vi "Local Test.vi"() -> ()   [LabVIEW 2021]
uses:
  Source/Omni-Bus/Omni_Bus.lvclass
  Source/Local Vars/Local Vars.lvclass
  Source/Omni-Bus/Support/Broad Types.ctl
  <vilib>/TSA/Abstract Data Classes/Constants/Support/U8/U8.vi
  <vilib>/TSA/Abstract Data Classes/Constants/Support/U8/Const_U8.lvclass
  <vilib>/TSA/Abstract Data Classes/Constants/Support/Str/Str.vi
  <vilib>/TSA/Abstract Data Classes/Constants/Support/Str/Const_Str.lvclass
  <vilib>/TSA/Abstract Data Classes/Constants/Support/DBL/DBL.vi
  <vilib>/TSA/Abstract Data Classes/Constants/Support/DBL/Const_DBL.lvclass
  <vilib>/TSA/Abstract Data Classes/Constants/Support/Bool/Bool.vi
  <vilib>/TSA/Abstract Data Classes/Constants/Support/Bool/Const_Bool.lvclass
  Source/Omni-Bus/Get/Static/Get Static Boolean.vi
  <vilib>/TSA/Abstract Data Classes/Abs_Types/Boolean/Static Read.vi
  <vilib>/TSA/Abstract Data Classes/Abs_Types/Boolean/Abs_Boolean.lvclass
  <vilib>/TSA/Abstract Data Classes/Abs_Types/Boolean/Static Write.vi
  C:/Program Files (x86)/National Instruments/LabVIEW 2021/vi.lib/TSA/Abstract Data Classes/Abs_Types/Value/Abs_Value.lvclass
  C:/Program Files (x86)/National Instruments/LabVIEW 2021/vi.lib/TSA/Abstract Data Classes/Abs_Types/Type/Abs_Type.lvclass
  C:/Program Files (x86)/National Instruments/LabVIEW 2021/vi.lib/TSA/Abstract Data Classes/Abs_Types/Boolean/Abs_Boolean.lvclass
  C:/Program Files (x86)/National Instruments/LabVIEW 2021/vi.lib/TSA/Abstract Data Classes/Abs_Types/Double Float/Abs_Double Float.lvclass
  C:/Program Files (x86)/National Instruments/LabVIEW 2021/vi.lib/TSA/Abstract Data Classes/Abs_Types/Floating Point/Abs_Floating Point.lvclass
  C:/Program Files (x86)/National Instruments/LabVIEW 2021/vi.lib/TSA/Abstract Data Classes/Abs_Types/Numeric/Abs_Numeric.lvclass
  C:/Program Files (x86)/National Instruments/LabVIEW 2021/vi.lib/TSA/Abstract Data Classes/Constants/Support/DBL/Const_DBL.lvclass
  C:/Program Files (x86)/National Instruments/LabVIEW 2021/vi.lib/TSA/Abstract Data Classes/Constants/Support/Interface/Const_Intf.lvclass
  <vilib>/TSA/Abstract Data Classes/Abs_Types/String/Abs_String.lvclass
  C:/Program Files (x86)/National Instruments/LabVIEW 2021/vi.lib/TSA/Abstract Data Classes/Abs_Types/String/Abs_String.lvclass
  C:/Program Files (x86)/National Instruments/LabVIEW 2021/vi.lib/TSA/Abstract Data Classes/Abs_Types/U8 Integer/Abs_U8 Integer.lvclass
  C:/Program Files (x86)/National Instruments/LabVIEW 2021/vi.lib/TSA/Abstract Data Classes/Abs_Types/Integer/Abs_Integer.lvclass
  C:/Program Files (x86)/National Instruments/LabVIEW 2021/vi.lib/TSA/Abstract Data Classes/Constants/Support/U8/Const_U8.lvclass
  <vilib>/TSA/Abstract Data Classes/Abs_Types/Value/Abs_Value.lvclass
  C:/Users/Tim/Documents/GitHub/VarBus/Source/Bus_Access/Bus_Access.lvclass
  C:/Users/Tim/Documents/GitHub/VarBus/Source/Local Vars/Local Vars.lvclass
  <vilib>/TSA/Abstract Data Classes/Abs_Types/Double Float/Support/Type.ctl
  <vilib>/TSA/Abstract Data Classes/Abs_Types/Double Float/Abs_Double Float.lvclass
panel:
  in  "Value 2":T1
  in  "stop 2":bool
  in  "stop":bool
  out "Value":T1
  out "Tags":string[](array[string])
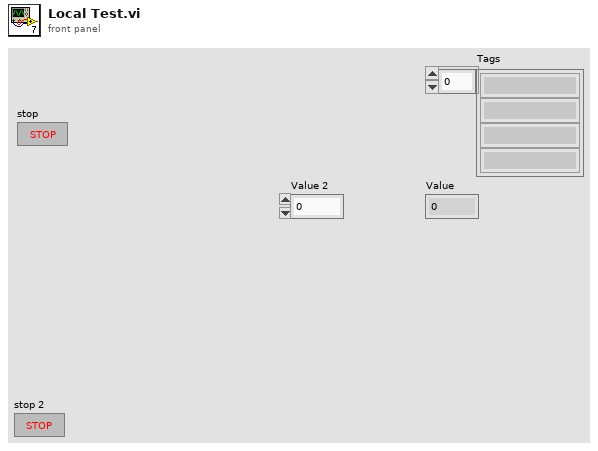
[diagram p1: front panel]
types:
  T1 = typedef "Abs_Double Float.lvclass/Type.ctl" = dbl
  T2 = typedef "Omni_Bus.lvclass/Broad Types.ctl" = enum16{"All Tags", "NI Specific Type", "Boolean", "String", "Numeric", "Float", "Integer", "Collection", "All Value Types", "Non Value Types"}
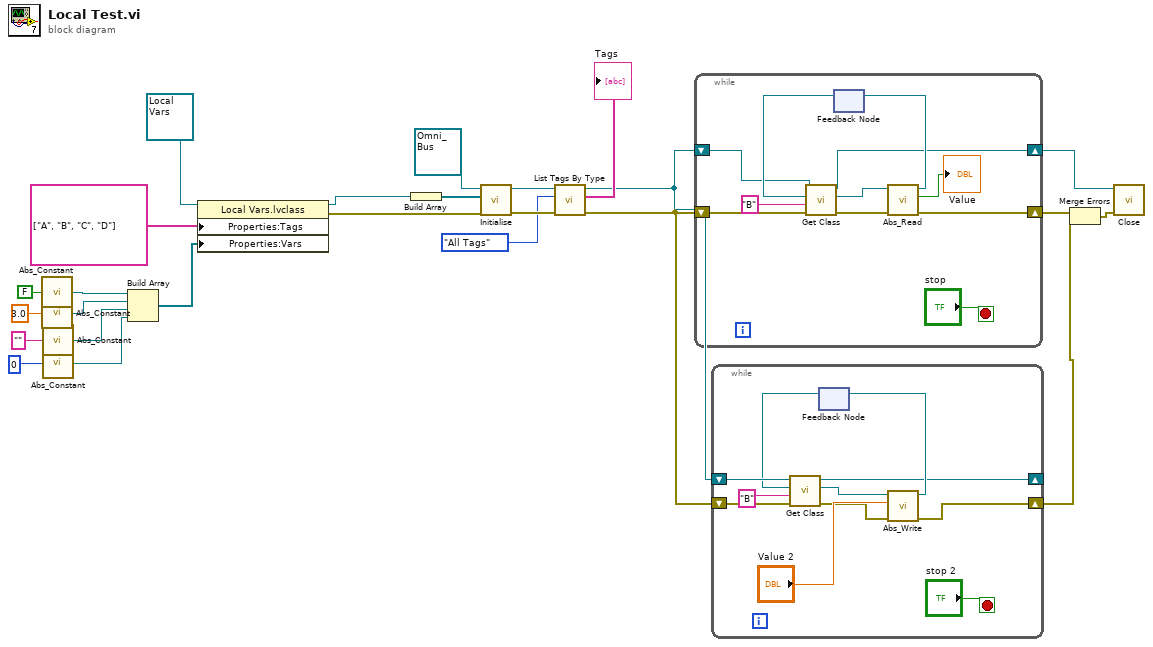
[diagram p0: block diagram]
diagram:
  n1 = call-poly <vilib>:"Abs_Constant.vi"("Boolean"=FALSE) -> ("Abs_Boolean.lvclass"=w19:refnum<class "Abs_Boolean.lvclass">)  [unwired: 4 in]
  n2 = call-poly <vilib>:"Abs_Constant.vi"("Value"=3.0) -> ("Constant"=w18:refnum<class "Const_DBL.lvclass">)  [unwired: 4 in]
  n3 = call-poly <vilib>:"Abs_Constant.vi"("String"="") -> ("Abs_String.lvclass"=w17:refnum<class "Abs_String.lvclass">)  [unwired: 4 in]
  n4 = call-poly <vilib>:"Abs_Constant.vi"("Value"=u8 0) -> ("Constant"=w9:refnum<class "Const_U8.lvclass">)  [unwired: 4 in]
  n5 = Build Array(w19, w18, w17, w9) -> (w14:refnum<class "Abs_Value.lvclass">[])
  n6 = property class="Local Vars.lvclass"(reference=refnum<class "Local Vars.lvclass"> refnum ("Data in"), "Properties:Tags"=string[] ["A", "B", "C", "D"] ("Tags"), "Properties:Vars"=w14) -> (reference out=w22:refnum<class "Local Vars.lvclass">, error out=w23:errorcluster)  [unwired: 1 in]
  n7 = Build Array(w22) -> (w24:refnum<class "Local Vars.lvclass">[])
  n8 = call-dynamic "Initialise.vi"("error in (no error)"=w23, "Var Access"=w24, "Var Bus in"=refnum<class "Omni_Bus.lvclass"> refnum) -> ("error out"=w12:errorcluster, "Var Bus out"=w13:refnum<class "Omni_Bus.lvclass">)  [unwired: 7 in]
  n9 = call-dynamic "List Tags By Type.vi"("error in (no error)"=w12, "Broad Types"=Broad_Types."All Tags", "Var Bus in"=w13) -> ("error out"=w3:errorcluster, "Tags"=→"Tags":string[], "Var Bus out"=w4:refnum<class "Omni_Bus.lvclass">)  [unwired: 5 in, 1 out]
  n10 = while {
    shift-right: [w26] -> w6
    shift-left: w4 -> [w29]
    shift-right: [w36] -> w5
    shift-left: w3 -> [w32]
    stop <- "stop" stop-if-true
    n11 = feedback #1() -> (w30:refnum<class "Abs_Boolean.lvclass">)  [unwired: 1 in]
    n12 = call-poly "Get Class.vi"("error in (no error)"=w32, "Tag"="B", "Value Type"=w30, "Var Bus in"=w29) -> ("error out"=w27:errorcluster, "Value Out"=w28:refnum<class "Abs_Boolean.lvclass">, "Var Bus out"=w26:refnum<class "Omni_Bus.lvclass">)  [unwired: 5 in]
    n13 = call-poly <vilib>:"Abs_Read.vi"("error in (no error)"=w27, "Abs_Boolean in"=w28) -> ("error out"=w36:errorcluster, "Boolean"=→"Value":bool, "Abs_Boolean out"=w33:refnum<class "Abs_Boolean.lvclass">)  [unwired: 7 in]
    n14 = feedback-in #1(w33) -> ()
  }
  n15 = while {
    shift-right: [w38] -> _
    shift-left: w4 -> [w43]
    shift-right: [w46] -> w1
    shift-left: w3 -> [w42]
    stop <- "stop 2" stop-if-true
    n16 = feedback #2() -> (w41:refnum<class "Abs_Boolean.lvclass">)  [unwired: 1 in]
    n17 = call-poly "Get Class.vi"("error in (no error)"=w42, "Tag"="B", "Value Type"=w41, "Var Bus in"=w43) -> ("error out"=w39:errorcluster, "Value Out"=w37:refnum<class "Abs_Boolean.lvclass">, "Var Bus out"=w38:refnum<class "Omni_Bus.lvclass">)  [unwired: 5 in]
    n18 = call-poly <vilib>:"Abs_Write.vi"("error in (no error)"=w39, "Boolean"="Value 2", "Abs_Boolean in"=w37) -> ("error out"=w46:errorcluster, "Abs_Boolean out"=w44:refnum<class "Abs_Boolean.lvclass">)  [unwired: 7 in]
    n19 = feedback-in #2(w44) -> ()
  }
  n20 = Merge Errors(w5, w1) -> (w2:errorcluster)
  n21 = call-dynamic "Close.vi"("error in (no error)"=w2, "Data in"=w6) -> ()  [unwired: 8 in, 2 out]
